vi "Propagate Abort Locally.vi"(8 "error in (no error)":errorcluster, 10 "New Abort Value":bool, 11 "Guardian in":refnum<class "Guardian.lvclass">) -> (0 "error out":errorcluster, 3 "Guardian out":refnum<class "Guardian.lvclass">)   [LabVIEW 2026, in "TALOS.lvlib" / "Guardian.lvlib" / "Guardian.lvclass"]
uses:
  Guardian.lvclass
  Guardian.lvclass/Guardian.ctl
  Classes/uService List/uService List.lvclass/uService List.ctl
  Father of all uServices/Father of all uServices/Event Handler Items.ctl
  builds/Actor Framework PPL/Actor Framework.lvlibp/1abvi3w/vi.lib/ActorFramework/Message Enqueuer/Message Priority.ctl
  Father of all uServices/Father of all uServices Messages/Event Handler Msg/Event Handler Msg.lvclass/Event Handler Msg.ctl
  Ancestor/Ancestor/Ancestor.lvclass/Ancestor.ctl
  Classes/uService List/Get all Queue.vi
  Support VIs/Generate Error.vi
  FGV/Error Memory/Get Error Description.vi
  Support VIs/Get PC name.vi
  Ancestor/Ancestor/Read ID.vi
  Support VIs/Get Class Name.vi
  <vilib>/Utility/error.llb/Clear Errors.vi
  FGV/Error Memory/Error Memory Core.vi
  <vilib>/AdvancedString/Delimited String to 1D String Array.vi
  <vilib>/AdvancedString/Delimited String to 1D String Array (string).vi
  Support VIs/Circus Root Path.vi
  FGV/Error Memory/Error Crt Lvl checker.vi
  FGV/Error Memory/Error Memory Core.vi/40c8088d-b597-4017-91af-faa98e00292e.vi
  FGV/Error Memory/Error Memory Core.vi/d4a3ab98-063c-4e44-b43d-fbdcfe6c2be2.vi
  builds/Actor Framework PPL/Actor Framework.lvlibp/1abvi3w/vi.lib/ActorFramework/Message Enqueuer/Enqueue.vi
  Support VIs/Global Memory.vi
  <vilib>/Utility/LVClass/Get LV Class Name.vi
  Support VIs/Is in Packed Library.vi
  Support VIs/TALOS Root path.vi
  Support VIs/Read CSV worksheet.vi
  Support VIs/Global Constants.vi
  <vilib>/Utility/error.llb/General Error Handler.vi
  Support VIs/Error Log.vi
  Father of all uServices/Father of all uServices Messages/Event Handler Msg/Event Handler Msg.lvclass
  Ancestor/Ancestor/Ancestor.lvclass
  <vilib>/Comparison/Equal/Equal Functor/Equal Functor.lvclass
  Classes/uService List/uService List.lvclass
  builds/Actor Framework PPL/Actor Framework.lvlibp/1abvi3w/vi.lib/ActorFramework/Message Enqueuer/Message Enqueuer.lvclass
  Father of all uServices/Father of all uServices/Father of all uServices.lvclass
  TALOS.lvlib
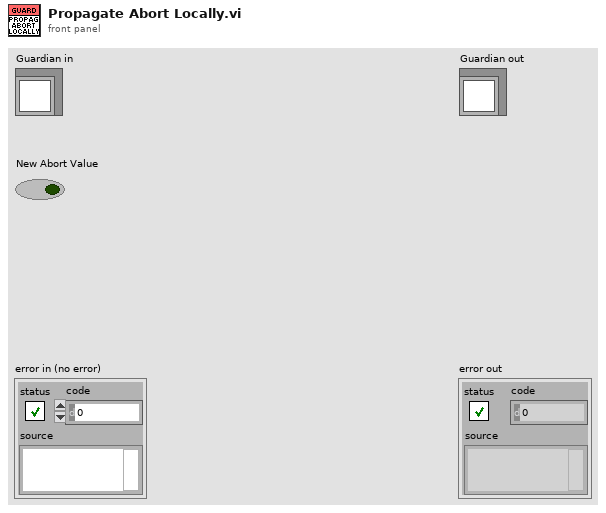
[diagram p1: front panel]
types:
  T1 = typedef "Actor Framework.lvlibp/Message Enqueuer.lvclass/Message Priority.ctl" = enum16{"Low", "Normal", "High"}
  T2 = typedef "TALOS.lvlib/Father of all uServices.lvlib/Father of all uServices.lvclass/Event Handler Items.ctl" = enum16{"Button Pressed", "Message", "Ready to launch?", "Safe Mode", "Start RUN", "Stop RUN"}
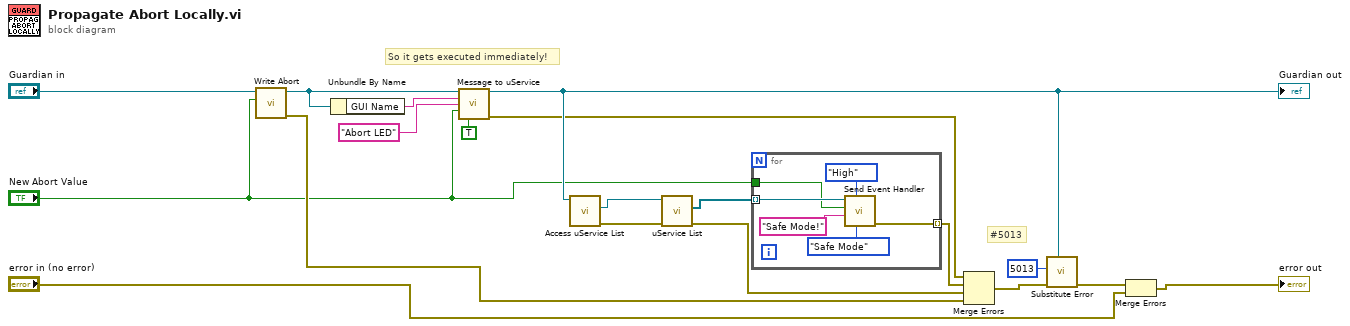
[diagram p0: block diagram]
diagram:
  # "#5013"
  # "So it gets executed immediately!"
  n1 = call "Write Abort.vi"("Abort value"="New Abort Value", "Guardian in"="Guardian in") -> ("error out"=w2:errorcluster, "Guardian out"=w5:refnum<class "Guardian.lvclass">)  [unwired: 8 in]
  n2 = Unbundle By Name(w5) -> ("GUI Name"=w13:string)
  n3 = call "Message to uService.vi"("Guardian in"=w5, "uService ID"=w13, "Message"="Abort LED", "Data"="New Abort Value", "Locale?"=TRUE) -> ("Guardian out"=w17:refnum<class "Guardian.lvclass">, "error out"=w15:errorcluster)  [unwired: 9 in]
  "Guardian out" <- w17
  n4 = call-dynamic "Access uService List.vi"("Ancestor in"=w17) -> ("error out"=w10:errorcluster, "uService List out"=w9:refnum<class "uService List.lvclass">)  [unwired: 8 in, 1 out]
  n5 = call-poly "uService List.vi"("error in (no error)"=w10, "uService List"=w9) -> ("error out"=w3:errorcluster, "All queues"=w11:refnum<class "Message Enqueuer.lvclass">[])  [unwired: 7 in, 1 out]
  n6 = for {
    tunnel: w11 -> [w24] mode=indexing
    tunnel: [w23] -> w4 mode=indexing
    tunnel: "New Abort Value" -> [w20]
    n7 = call "Send Event Handler.vi"("Event type"=Event_Handler_Items."Safe Mode", "Message Priority (Normal)"=Message_Priority."High", "Item Name"="Safe Mode!", "Data"=w20, "Message Enqueuer"=w24) -> ("error out"=w23:errorcluster)  [unwired: 5 in, 1 out]
  }
  n8 = Merge Errors(w15, w4, w3, w2) -> (w8:errorcluster)
  n9 = call "Substitute Error.vi"("LabVIEW Object"=w17, "error in (no error)"=w8, "Error Code"=5013) -> ("error out"=w16:errorcluster)  [unwired: 8 in]
  n10 = Merge Errors(w16, "error in (no error)") -> (→"error out":errorcluster)
